vi "UI_Start Asychronous Call.vi"(8 "error in (no error)":errorcluster, 9 "String":string, 10 "VI Refnum":refnum<vi>, 11 "User Event in":refnum<user-event>) -> (0 "error out":errorcluster, 3 "VI out":refnum<vi>)   [LabVIEW 2025]
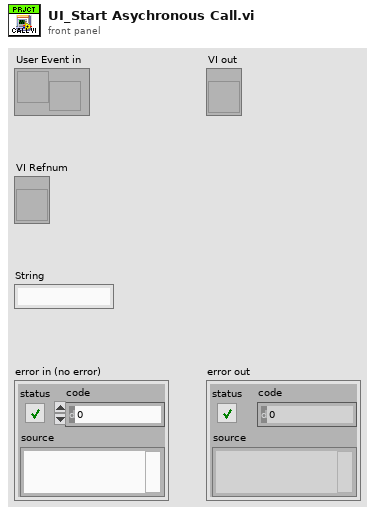
[diagram p1: front panel]
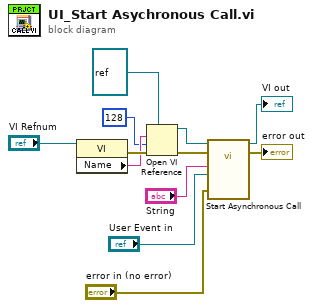
[diagram p0: block diagram]
diagram:
  n1 = property class="VI"(reference="VI Refnum") -> (error out=w7:errorcluster, "Name"=w3:string)  [unwired: 1 in, 1 out]
  n2 = Open VI Reference(type specifier VI Refnum (for type only)=refnum<vi> refnum, vi path=w3, options=128, error in (no error)=w7) -> (vi reference=w5:refnum<vi>, error out=w6:errorcluster)  [unwired: 2 in]
  n3 = call-by-ref "Start Asynchronous Call"(reference=w5, error in=w6, 8:"error in (no error)"="error in (no error)", "event source"="User Event in", "String"="String") -> (reference out=→"VI out":refnum<vi>, error out=→"error out":errorcluster)  [unwired: 8 in, 1 out]
